vi "ep_Check Delta Order.vi"(8 "error in (no error)":errorcluster, 11 "delta order":dbl[](array[numeric])) -> (0 "error out":errorcluster, 3 "cycles per block":i32)   [LabVIEW 2013, in "NI_EP_Power Measurement.lvlib"]
uses:
  <vilib>/addons/Electrical Power/Power Measurement/NI_EP_Power Measurement.lvlib
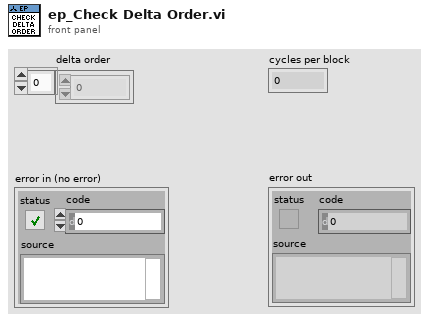
[diagram p1: front panel]
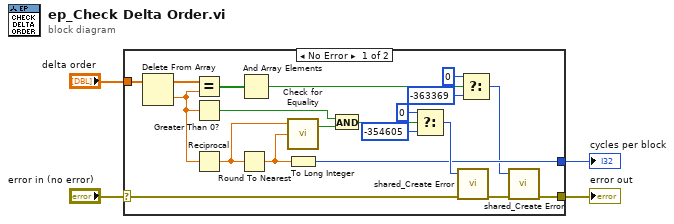
[diagram p0: block diagram]
diagram:
  n1 = case shown="No Error" "error in (no error)" {
    selector: "error in (no error)" -> [w13 w25]
    tunnel: "delta order" -> [w23 _]
    tunnel: [w9 w25] -> w3
    tunnel: [w15 _] -> w2
    frame No Error {
      n2 = Delete From Array(array=w23) -> (deleted portion=w14:dbl, array with subset deleted=w22:dbl[])  [unwired: 2 in]
      n3 = Equal?(x=w22, y=w14) -> (x = y?=w21:bool[])
      n4 = Greater Than 0?(x=w14) -> (x > 0?=w12:bool)
      n5 = Reciprocal(x=w14) -> (1/x=w24:dbl)
      n6 = Round To Nearest(number=w24) -> (nearest integer value=w16:dbl)
      n7 = And Array Elements(Boolean array=w21) -> (logical AND=w6:bool)
      n8 = call <vilib>:"Check for Equality.vi"("n2"=w16, "n1"=w24) -> ("equal?"=w11:bool)  [unwired: 1 in, 1 out]
      n9 = To Long Integer(number=w16) -> (32bit integer=w15:i32)
      n10 = And(x=w12, y=w11) -> (x .and. y?=w20:bool)
      n11 = Select(t=0, s=w20, f=-354605) -> (s? t:f=w17:i32)
      n12 = call <vilib>:"shared_Create Error.vi"("error in (no error)"=w13, "error code (0)"=w17) -> ("error out"=w10:errorcluster)  [unwired: 9 in]
      n13 = Select(t=0, s=w6, f=-363369) -> (s? t:f=w5:i32)
      n14 = call <vilib>:"shared_Create Error.vi"("error in (no error)"=w10, "error code (0)"=w5) -> ("error out"=w9:errorcluster)  [unwired: 9 in]
    }
    frame Error {
    }
  }
  "error out" <- w3
  "cycles per block" <- w2
